vi "ASK_DeModulation.vi"(5 "rx_data":cdb[](array[numeric]), 8 "error in (no error)":errorcluster caption="错误输入（无错误）", 11 "PathIn":path) -> (0 "error out":errorcluster caption="错误输出", 3 "PathOut":path, 6 "data":dbl[](array[numeric]))   [LabVIEW 2015]
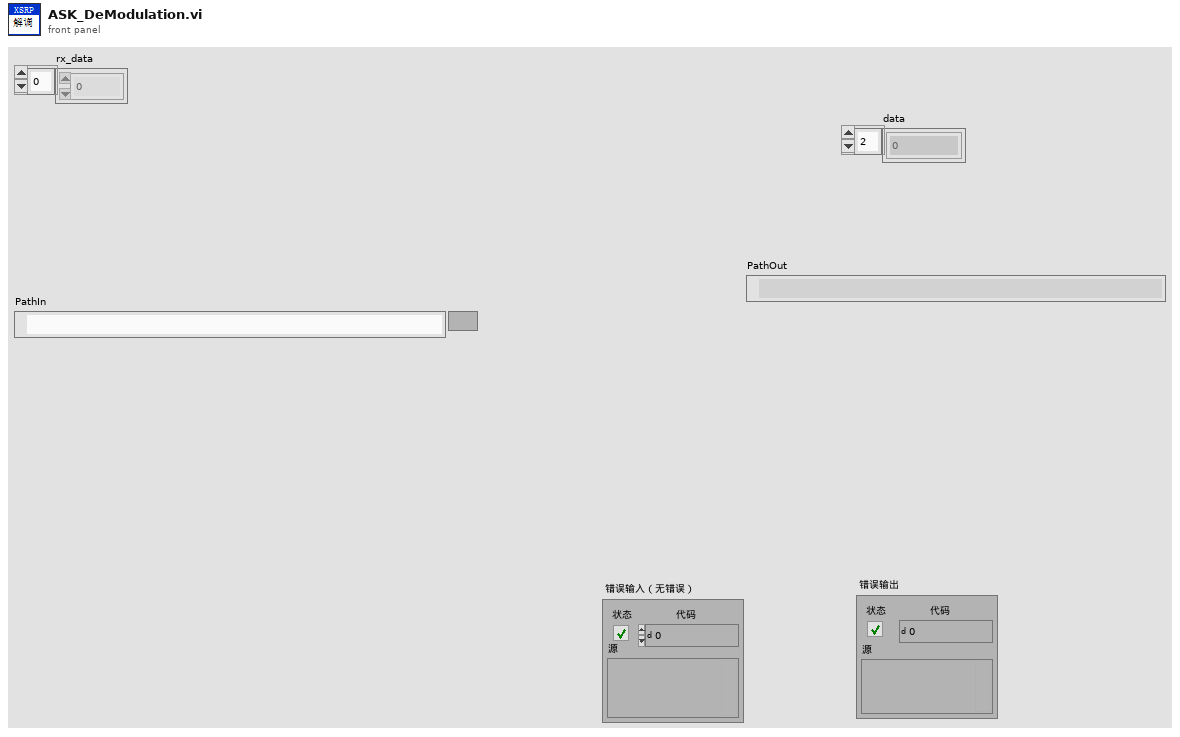
[diagram p1: front panel]
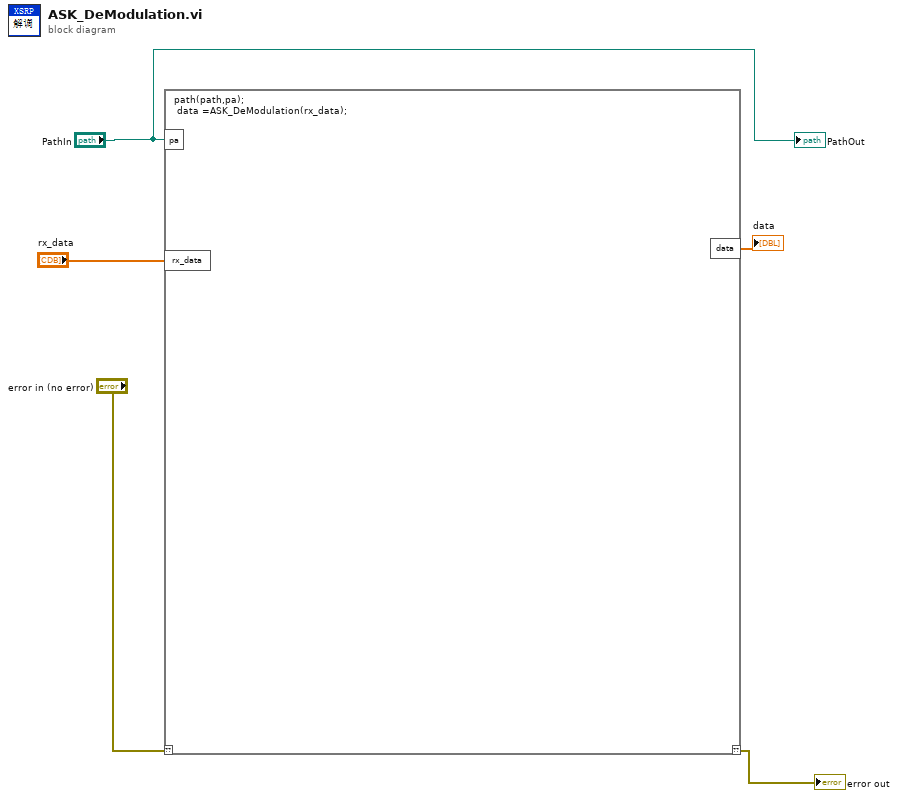
[diagram p0: block diagram]
diagram:
  n1 = script code="path(path,pa);\n data =ASK_DeModulation(rx_data);"("??"="error in (no error)", "pa"="PathIn", "rx_data"="rx_data") -> ("??"=→"error out":errorcluster, "data"=→"data":dbl[])
  "PathOut" <- "PathIn"
